vi "Vision Processing.vi"(4 "error in (no error)":errorcluster, 7 "Image Size":T1=enum."320x240") -> ()   [LabVIEW 2019]
doc: "This VI runs in parallel to other tasks. It gets images from the camera, processes them for color or shape and use that information to affect robot behavior."
uses:
  <vilib>/Rock Robotics/WPI/Camera/WPI_CameraImageSize.ctl
  <vilib>/Rock Robotics/WPI/Camera/WPI_CameraWhite Balance Values.ctl
  <vilib>/Rock Robotics/WPI/Camera/WPI_CameraExposure Values.ctl
  <vilib>/Rock Robotics/WPI/Camera/WPI_CameraFrameRate.ctl
  Robot Global Data.vi
panel:
  in  "Image Size 2":T1=enum."320x240"
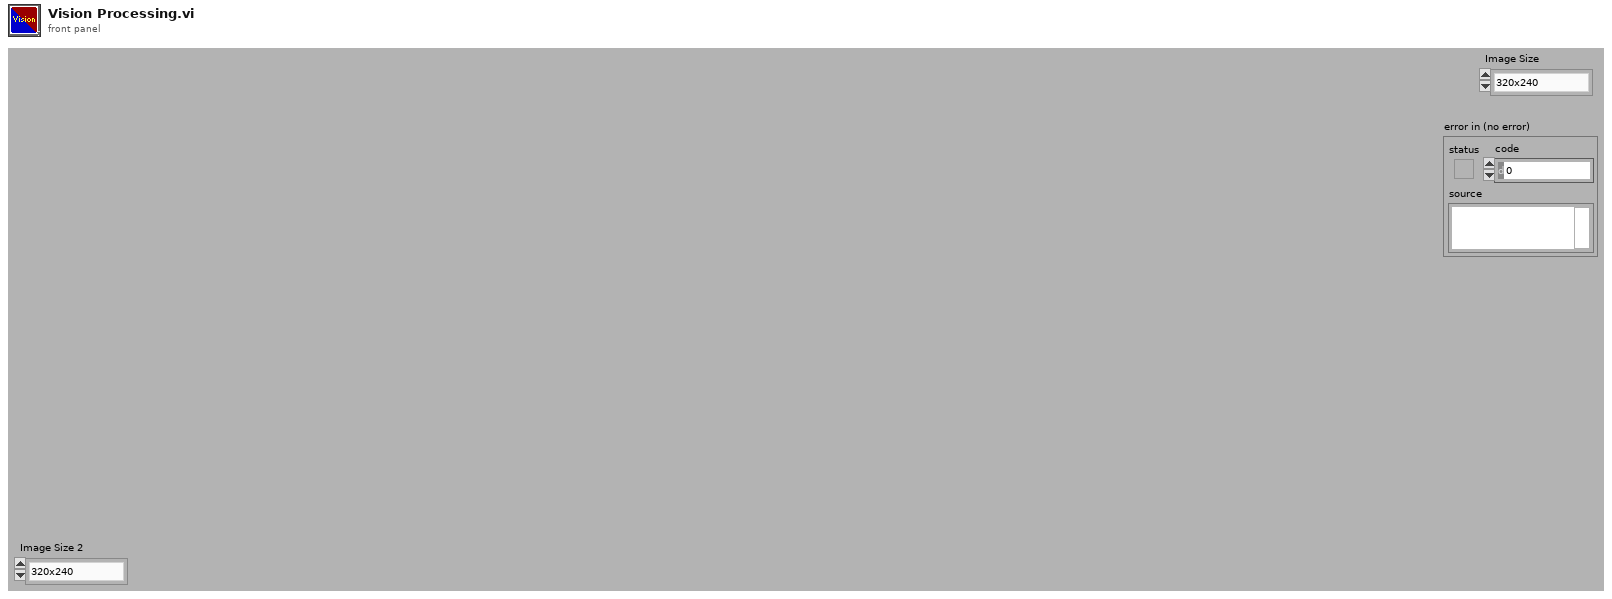
[diagram p1: front panel]
types:
  T1 = typedef "WPI_CameraImageSize.ctl" = enum16{"640x480", "320x240", "160x120", "Custom"}
  T2 = typedef "WPI_CameraFrameRate.ctl" = u32
  T3 = typedef "WPI_CameraExposure Values.ctl" = enum16{"Auto", "Flicker-free 50 Hz", "Flicker-free 60 Hz", "Hold current", "Custom"}
  T4 = typedef "WPI_CameraWhite Balance Values.ctl" = enum16{"Auto", "Fixed indoor", "Fixed outdoor 1", "Fixed outdoor 2", "Fixed fluorescent 1", "Fixed fluorescent 2", "Hold current", "Custom"}
  T5 = typedef "Image Type" = u32
  T6 = typedef "WPI_CameraDevRef.ctl" = cluster{"Camera Address":string, "CameraStatus":errorcluster}
  T7 = typedef "IMAQ Image.ctl" = refnum<image>
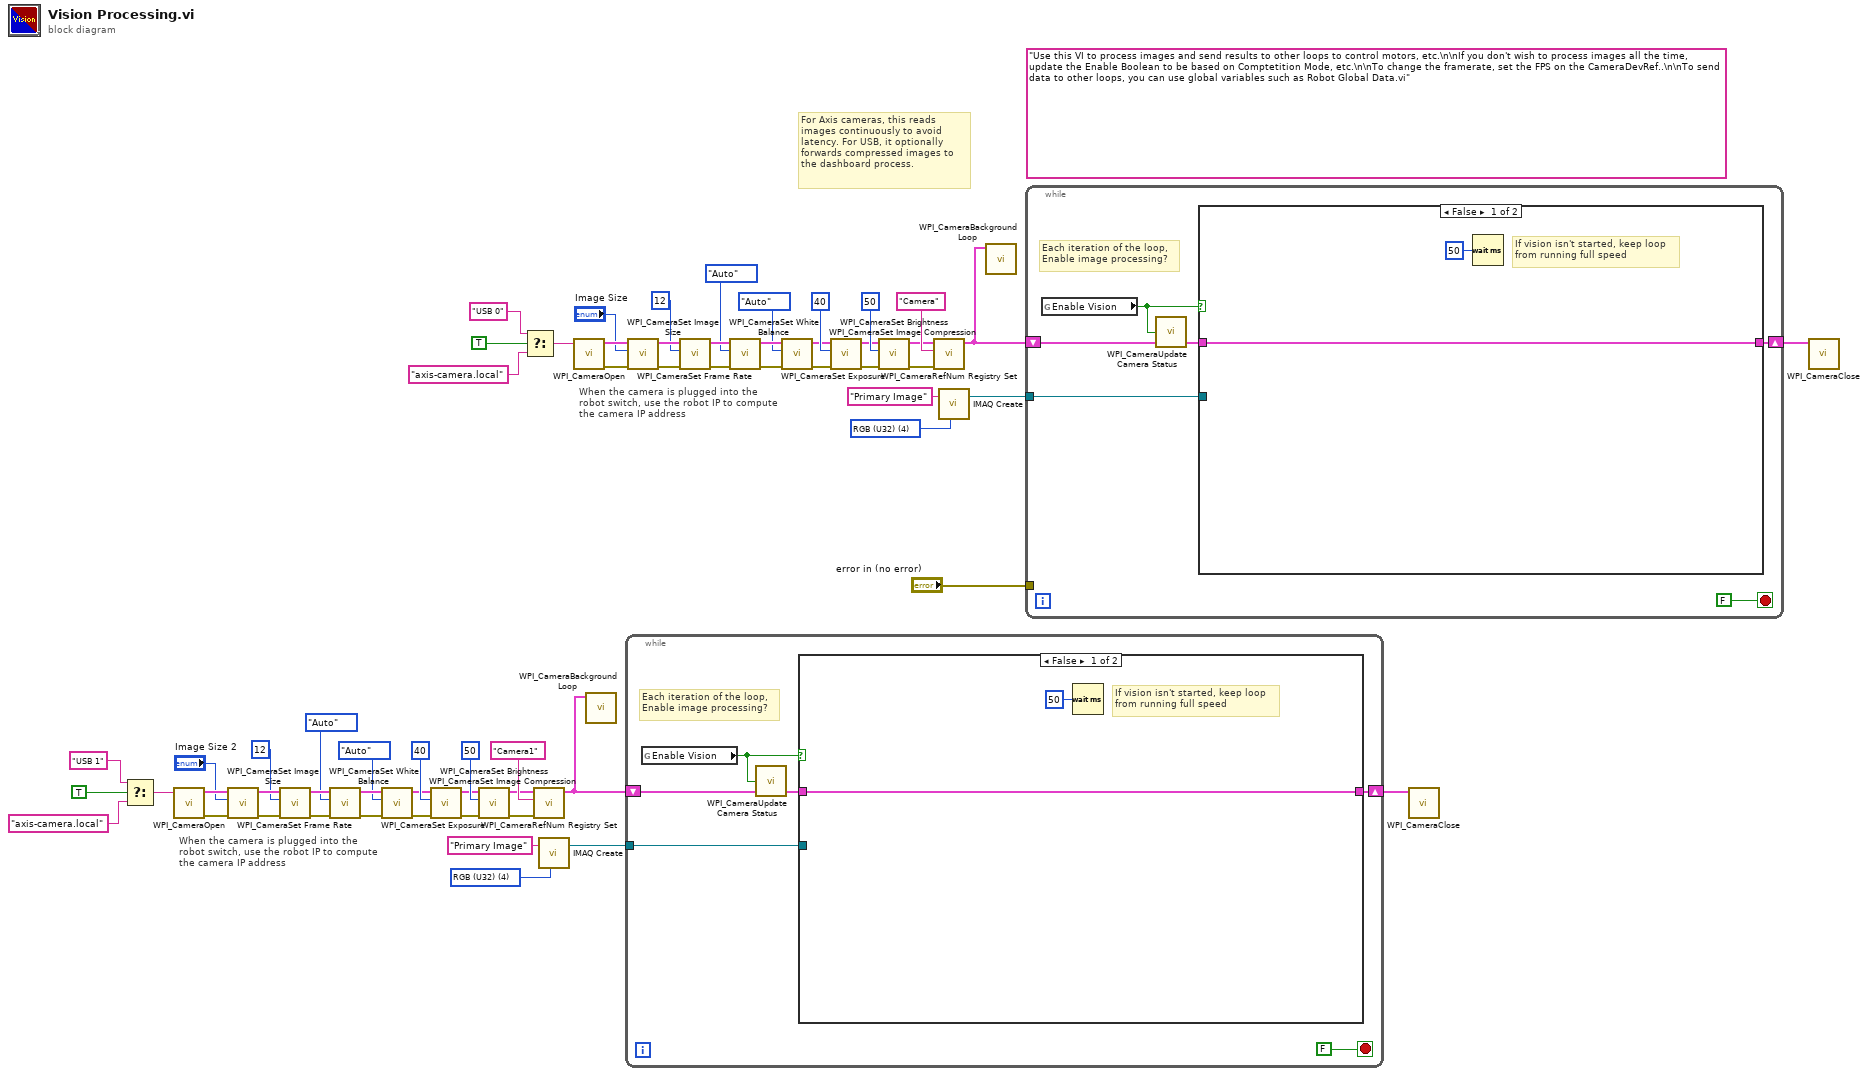
[diagram p0: block diagram]
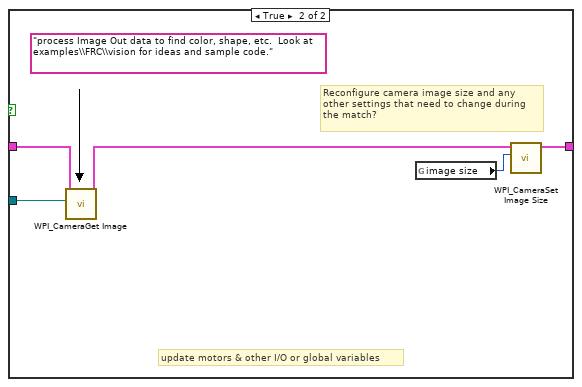
[diagram p2: hidden frame]
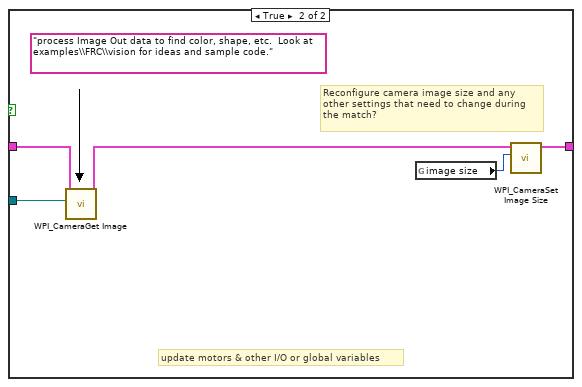
[diagram p3: hidden frame]
diagram:
  w30 = T5 4 items=["Grayscale (U8)", "Grayscale (I16)", "Grayscale (SGL)", "Complex (CSG)", "RGB (U32)", "HSL (U32)", "RGB (U64)"] ("Image Type")
  (unwired) "Use this VI to process images and send results to other loops to control motors, etc.\n\nIf you don't wish to process images all the time, update the Enable Boolean to be based on Comptetition Mode, etc.\n\nTo change the framerate, set the FPS on the CameraDevRef..\n\nTo send data to other loops, you can use global variables such as Robot Global Data.vi"
  w61 = T5 4 items=["Grayscale (U8)", "Grayscale (I16)", "Grayscale (SGL)", "Complex (CSG)", "RGB (U32)", "HSL (U32)", "RGB (U64)"] ("Image Type")
  # "When the camera is plugged into the\nrobot switch, use the robot IP to compute\nthe camera IP address"
  # "When the camera is plugged into the\nrobot switch, use the robot IP to compute\nthe camera IP address"
  # "For Axis cameras, this reads\nimages continuously to avoid\nlatency. For USB, it optionally\nforwards compressed images to\nthe dashboard process."
  n1 = Select(t="USB 1" ("format string"), s=TRUE ("dot notation? (F)"), f="axis-camera.local" ("format string")) -> (s? t:f=w2:string)
  n2 = call <vilib>:"WPI_CameraOpen.vi"("Camera Address"=w2) -> ("error out"=w18:errorcluster, "CameraDevRef"=w19:T6)  [unwired: 1 in, 8 out]
  n3 = call <vilib>:"WPI_CameraSet Image Size.vi"("error in (no error)"=w18, "Image Size"="Image Size 2", "CameraDevRef"=w19) -> ("error out"=w17:errorcluster, "CameraDevRef Out"=w20:T6)  [unwired: 1 in, 6 out]
  n4 = call <vilib>:"WPI_CameraSet Frame Rate.vi"("error in (no error)"=w17, "Frame Rate (fps)"=T2 12, "CameraDevRef"=w20) -> ("error out"=w16:errorcluster, "CameraDevRef Out"=w22:T6)  [unwired: 7 out]
  n5 = call <vilib>:"WPI_CameraSet White Balance.vi"("error in (no error)"=w16, "White Balance"=WPI_CameraWhite_Balance_Values."Auto", "CameraDevRef"=w22) -> ("error out"=w15:errorcluster, "CameraDevRef Out"=w21:T6)  [unwired: 1 in, 6 out]
  n6 = call <vilib>:"WPI_CameraSet Exposure.vi"("error in (no error)"=w15, "Exposure"=WPI_CameraExposure_Values."Auto", "CameraDevRef"=w21) -> ("error out"=w14:errorcluster, "CameraDevRef Out"=w24:T6)  [unwired: 1 in, 6 out]
  n7 = call <vilib>:"WPI_CameraSet Image Compression.vi"("error in (no error)"=w14, "Compression"=40, "CameraDevRef"=w24) -> ("error out"=w13:errorcluster, "CameraDevRef Out"=w23:T6)  [unwired: 7 out]
  n8 = call <vilib>:"WPI_CameraSet Brightness.vi"("error in (no error)"=w13, "Brightness"=50, "CameraDevRef"=w23) -> ("error out"=w11:errorcluster, "CameraDevRef Out"=w12:T6)  [unwired: 1 in, 6 out]
  n9 = Select(t="USB 0" ("format string"), s=TRUE ("dot notation? (F)"), f="axis-camera.local" ("format string")) -> (s? t:f=w32:string)
  n10 = call <vilib>:"WPI_CameraRefNum Registry Set.vi"("error in (no error)"=w11, "refnum name"="Camera1", "CameraDevRef"=w12) -> ("CameraDevRef"=w7:T6)  [unwired: 1 in, 7 out]
  n11 = call "IMAQ Create"("Image Name"="Primary Image", "Image Type"=w30) -> ("New Image"=w28:T7)  [unwired: 2 in, 2 out]
  n12 = call <vilib>:"WPI_CameraOpen.vi"("Camera Address"=w32) -> ("error out"=w49:errorcluster, "CameraDevRef"=w50:T6)  [unwired: 1 in, 8 out]
  n13 = call <vilib>:"WPI_CameraBackground Loop.vi"("CameraDevRef"=w7) -> ()  [unwired: 11 in]
  n14 = while {
    shift-right: [w66] -> w5
    shift-left: w7 -> [w64]
    tunnel: w28 -> [w65]
    stop <- FALSE stop-if-true
    # "Each iteration of the loop,\nEnable image processing?"
    n15 = global read "Robot Global Data.vi" "Enable Vision"() -> (w62:bool)
    n16 = call <vilib>:"WPI_CameraUpdate Camera Status.vi"("CameraDevRef In"=w64, "Enable Vision"=w62) -> ("CameraDevRef Out"=w63:T6)  [unwired: 3 in]
    n17 = case shown="False" w62 {
      tunnel: w65 -> [_ w73]
      tunnel: [w69 w74] -> w66
      tunnel: w63 -> [w69 w71]
      frame False {
        # "If vision isn't started, keep loop\nfrom running full speed"
        n18 = Wait (ms)(milliseconds to wait=u32 50) -> ()  [unwired: 1 out]
      }
      frame True {
        (unwired) "process Image Out data to find color, shape, etc.  Look at examples\\FRC\\vision for ideas and sample code."
        # "update motors & other I/O or global variables"
        # "Reconfigure camera image size and any\nother settings that need to change during\nthe match?"
        n19 = call <vilib>:"WPI_CameraGet Image.vi"("Image"=w73, "CameraDevRef"=w71) -> ("CameraDevRef Out"=w70:T6)  [unwired: 1 in, 8 out]
        n20 = global read "Robot Global Data.vi" "image size"() -> (w72:T1)
        n21 = call <vilib>:"WPI_CameraSet Image Size.vi"("Image Size"=w72, "CameraDevRef"=w70) -> ("CameraDevRef Out"=w74:T6)  [unwired: 2 in, 7 out]
      }
    }
  }
  n22 = call <vilib>:"WPI_CameraSet Image Size.vi"("error in (no error)"=w49, "Image Size"="Image Size", "CameraDevRef"=w50) -> ("error out"=w48:errorcluster, "CameraDevRef Out"=w51:T6)  [unwired: 1 in, 6 out]
  n23 = call <vilib>:"WPI_CameraSet Frame Rate.vi"("error in (no error)"=w48, "Frame Rate (fps)"=T2 12, "CameraDevRef"=w51) -> ("error out"=w47:errorcluster, "CameraDevRef Out"=w53:T6)  [unwired: 7 out]
  n24 = call <vilib>:"WPI_CameraSet White Balance.vi"("error in (no error)"=w47, "White Balance"=WPI_CameraWhite_Balance_Values."Auto", "CameraDevRef"=w53) -> ("error out"=w46:errorcluster, "CameraDevRef Out"=w52:T6)  [unwired: 1 in, 6 out]
  n25 = call <vilib>:"WPI_CameraSet Exposure.vi"("error in (no error)"=w46, "Exposure"=WPI_CameraExposure_Values."Auto", "CameraDevRef"=w52) -> ("error out"=w45:errorcluster, "CameraDevRef Out"=w55:T6)  [unwired: 1 in, 6 out]
  n26 = call <vilib>:"WPI_CameraSet Image Compression.vi"("error in (no error)"=w45, "Compression"=40, "CameraDevRef"=w55) -> ("error out"=w44:errorcluster, "CameraDevRef Out"=w54:T6)  [unwired: 7 out]
  n27 = call <vilib>:"WPI_CameraSet Brightness.vi"("error in (no error)"=w44, "Brightness"=50, "CameraDevRef"=w54) -> ("error out"=w42:errorcluster, "CameraDevRef Out"=w43:T6)  [unwired: 1 in, 6 out]
  n28 = call <vilib>:"WPI_CameraRefNum Registry Set.vi"("error in (no error)"=w42, "refnum name"="Camera", "CameraDevRef"=w43) -> ("CameraDevRef"=w38:T6)  [unwired: 1 in, 7 out]
  n29 = call "IMAQ Create"("Image Name"="Primary Image", "Image Type"=w61) -> ("New Image"=w59:T7)  [unwired: 2 in, 2 out]
  n30 = call <vilib>:"WPI_CameraBackground Loop.vi"("CameraDevRef"=w38) -> ()  [unwired: 11 in]
  n31 = while {
    shift-right: [w79] -> w36
    shift-left: w38 -> [w77]
    tunnel: w59 -> [w78]
    tunnel: "error in (no error)" -> [_]
    stop <- FALSE stop-if-true
    # "Each iteration of the loop,\nEnable image processing?"
    n32 = global read "Robot Global Data.vi" "Enable Vision"() -> (w75:bool)
    n33 = call <vilib>:"WPI_CameraUpdate Camera Status.vi"("CameraDevRef In"=w77, "Enable Vision"=w75) -> ("CameraDevRef Out"=w76:T6)  [unwired: 3 in]
    n34 = case shown="False" w75 {
      tunnel: w78 -> [_ w86]
      tunnel: [w82 w87] -> w79
      tunnel: w76 -> [w82 w84]
      frame False {
        # "If vision isn't started, keep loop\nfrom running full speed"
        n35 = Wait (ms)(milliseconds to wait=u32 50) -> ()  [unwired: 1 out]
      }
      frame True {
        (unwired) "process Image Out data to find color, shape, etc.  Look at examples\\FRC\\vision for ideas and sample code."
        # "update motors & other I/O or global variables"
        # "Reconfigure camera image size and any\nother settings that need to change during\nthe match?"
        n36 = call <vilib>:"WPI_CameraGet Image.vi"("Image"=w86, "CameraDevRef"=w84) -> ("CameraDevRef Out"=w83:T6)  [unwired: 1 in, 8 out]
        n37 = global read "Robot Global Data.vi" "image size"() -> (w85:T1)
        n38 = call <vilib>:"WPI_CameraSet Image Size.vi"("Image Size"=w85, "CameraDevRef"=w83) -> ("CameraDevRef Out"=w87:T6)  [unwired: 2 in, 7 out]
      }
    }
  }
  n39 = call <vilib>:"WPI_CameraClose.vi"("CameraDevRef"=w5) -> ()  [unwired: 1 in, 10 out]
  n40 = call <vilib>:"WPI_CameraClose.vi"("CameraDevRef"=w36) -> ()  [unwired: 1 in, 10 out]
